vi "StandAloneApp_old.vi"() -> ()   [LabVIEW 2016]
panel:
  in  "Code 3":string
  in  "Code 2":string="# write code here\n"
  in  "Code 1":string="'''\nThis example will make SPIKE smile.\n\nIt is a good getting started example\n'''\n\nimport hub   # allows you to use all the SPIKE specific comands\n\nhub.display.show(hub.Image.SMILE)   # display a smile\n\n# for more examples on using the display, select the help button and look at the SPIKE examples\n"
  in  "Tab Control":enum32{"IntroPage", "Choose", "Examples"}(tab)
  in  "MoveOn":bool
  in  "Examples":bool
  in  "Blank":bool
  in  "W1.1 2":cluster{"Window Name":string, "Window1":bool}={"Window Name"="Select", "Window1"=FALSE}
  in  "W1.1 3":cluster{"Window Name":string, "Window1":bool}={"Window Name"="Select", "Window1"=FALSE}
  in  "W1.1":cluster{"Window Name":string, "Window1":bool}={"Window Name"="Select", "Window1"=FALSE}
  in  "Connections":enum32{"window 1", "window 2", "window 3"}(tab)
  in  "Device 3":bool
  in  "Device 2":bool
  in  "Device 1":bool
  in  "# Devices":enum32{"Page 1", "Page 2", "Page 3"}(tab)
  out "Description":string="This example will make SPIKE smile.\n\nIt is a good getting started example"
  out "Name":string="Smile"
  out "image":picture
  in  "Open Example":bool
  in  "Listbox":i32(listbox)
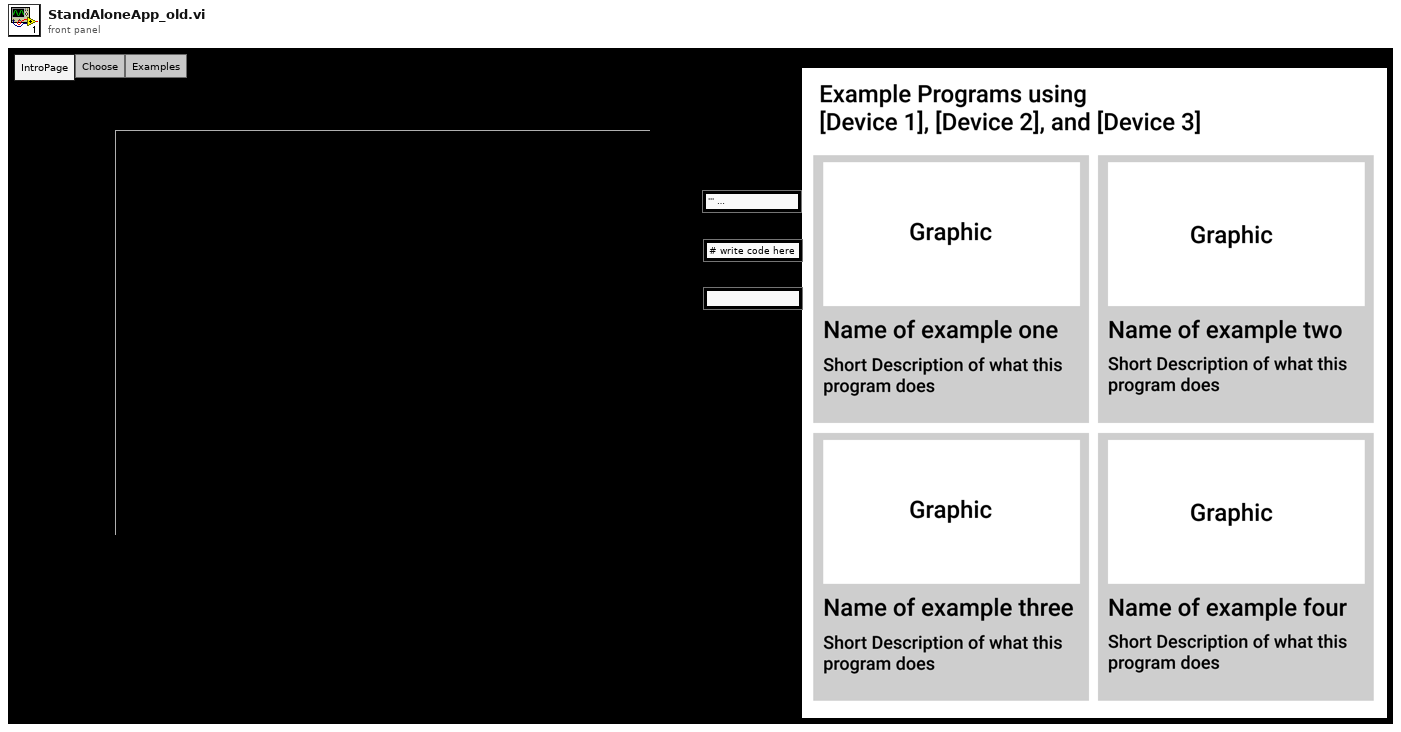
[diagram p1: front panel]
types:
  T1 = enum32{"Invalid", "Standard", "Closed", "Hidden", "Minimized", "Maximized"}
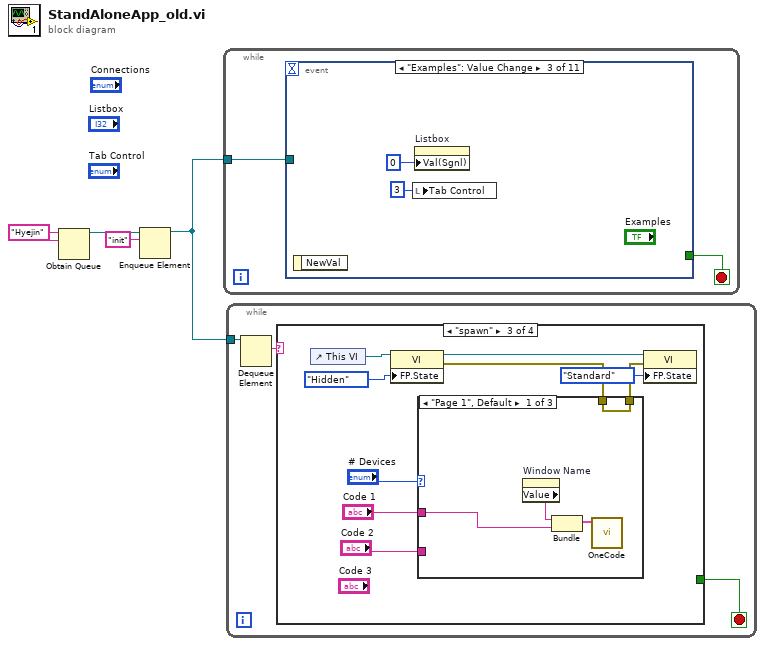
[diagram p0: block diagram]
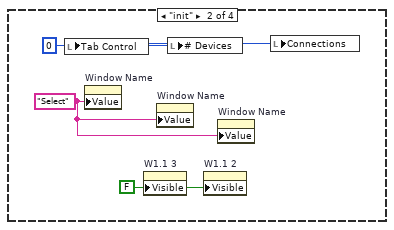
[diagram p3: hidden frame]
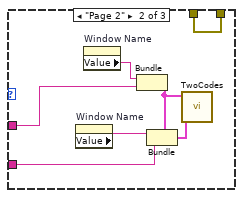
[diagram p4: hidden frame]
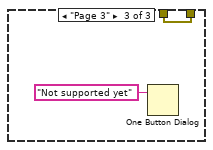
[diagram p5: hidden frame]
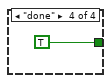
[diagram p6: hidden frame]
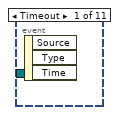
[diagram p7: hidden frame]
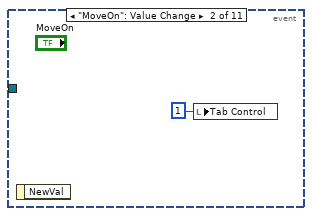
[diagram p8: hidden frame]
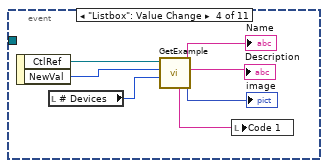
[diagram p9: hidden frame]
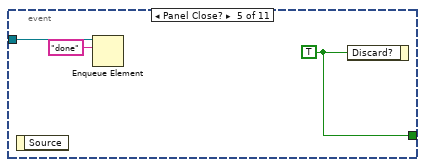
[diagram p10: hidden frame]
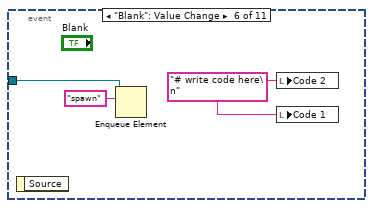
[diagram p11: hidden frame]
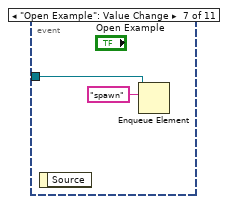
[diagram p12: hidden frame]
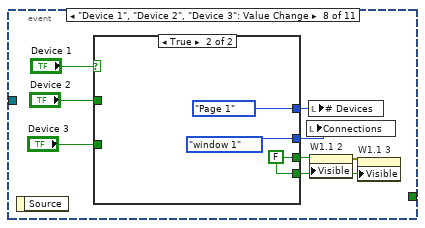
[diagram p13: hidden frame]
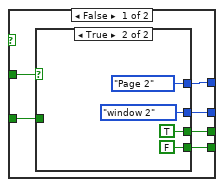
[diagram p14: hidden frame]
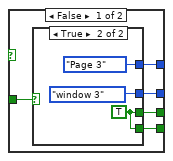
[diagram p15: hidden frame]
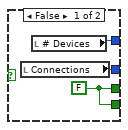
[diagram p16: hidden frame]
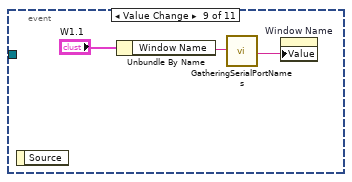
[diagram p17: hidden frame]
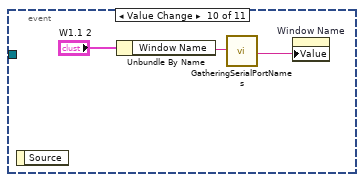
[diagram p18: hidden frame]
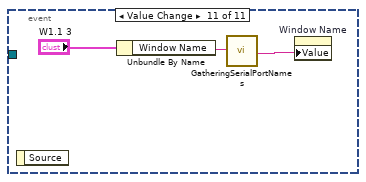
[diagram p19: hidden frame]
diagram:
  w1 = "Hyejin" ("name (unnamed)")
  n1 = Obtain Queue(name (unnamed)=w1, element data type=w1) -> (queue out=w4:refnum<queue>)  [unwired: 3 in, 2 out]
  n2 = Enqueue Element(queue=w4, element="init") -> (queue out=w2:refnum<queue>)  [unwired: 2 in, 2 out]
  n3 = while {
    tunnel: w2 -> [w5]
    stop <- w6 stop-if-true
    n4 = event shown="[2] \"Examples\": Value Change" {
      selector: _ -> [_ _ _ _ _ _ _ _ _ _ _]
      dyn-events: _ -> [_ _ _ _ _ _ _ _ _ _ _]
      timeout: _ -> [_ _ _ _ _ _ _ _ _ _ _]
      tunnel: [_ _ _ _ w19 _ _ _ _ _ _] -> w6
      tunnel: w5 -> [_ _ _ _ w17 w21 w23 _ _ _ _]
      event Timeout {
        n5 = event-data() -> ()  [unwired: 1 in, 3 out]
      }
      event "MoveOn": Value Change {
        n6 = event-data() -> ()  [unwired: 1 in, 1 out]
        n7 = local write "Tab Control"(1) -> ()
      }
      event "Examples": Value Change {
        n8 = event-data() -> ()  [unwired: 1 in, 1 out]
        n9 = local write "Tab Control"(3) -> ()
        n10 = property on="Listbox" class="LstBox (strict)"("Val(Sgnl)"=0 ("Listbox")) -> ()  [unwired: 2 in, 2 out]
      }
      event "Listbox": Value Change {
        n11 = event-data() -> ("CtlRef"=w15:refnum<vi>, "NewVal"=w14:i32)  [unwired: 1 in]
        n12 = local read "# Devices"() -> (w16:enum32{"Page 1", "Page 2", "Page 3"})
        n13 = call "GetExample.vi"("# Devices"=w16, "Listbox"=w14, "ListBox in"=w15) -> ("image"=→"image":picture, "description"=→"Description":string, "name"=→"Name":string, "Python"=w10:string)  [unwired: 5 in]
        n14 = local write "Code 1"(w10) -> ()
      }
      event Panel Close? {
        w19 = TRUE ("Discard?")
        n15 = event-data() -> ()  [unwired: 1 in, 1 out]
        n16 = Enqueue Element(queue=w17, element="done") -> ()  [unwired: 2 in, 3 out]
        n17 = event-data("Discard?"=w19) -> ()  [unwired: 1 in, 1 out]
      }
      event "Blank": Value Change {
        w20 = "# write code here\n" ("Code 2")
        n18 = event-data() -> ()  [unwired: 1 in, 1 out]
        n19 = Enqueue Element(queue=w21, element="spawn") -> ()  [unwired: 2 in, 3 out]
        n20 = local write "Code 2"(w20) -> ()
        n21 = local write "Code 1"(w20) -> ()
      }
      event "Open Example": Value Change {
        n22 = event-data() -> ()  [unwired: 1 in, 1 out]
        n23 = Enqueue Element(queue=w23, element="spawn") -> ()  [unwired: 2 in, 3 out]
      }
      event "Device 1", "Device 2", "Device 3": Value Change {
        n24 = event-data() -> ()  [unwired: 1 in, 1 out]
        n25 = case shown="True" "Device 1" {
          tunnel: [w38 enum32{"Page 1", "Page 2", "Page 3"}."Page 1" ("# Devices")] -> w32
          tunnel: "Device 2" -> [w37 _]
          tunnel: "Device 3" -> [w36 _]
          tunnel: [w35 enum32{"window 1", "window 2", "window 3"}."window 1" ("Connections 2")] -> w28
          tunnel: [w34 w54] -> w26
          tunnel: [w33 w54] -> w25
          frame False {
            n26 = case shown="True" w37 {
              tunnel: [w43 enum32{"Page 1", "Page 2", "Page 3"}."Page 2" ("# Devices")] -> w38
              tunnel: w36 -> [w42 _]
              tunnel: [w41 enum32{"window 1", "window 2", "window 3"}."window 2" ("Connections 2")] -> w35
              tunnel: [w40 TRUE ("Visible")] -> w34
              tunnel: [w39 FALSE ("Visible")] -> w33
              frame False {
                n27 = case shown="True" w42 {
                  tunnel: [w46 enum32{"Page 1", "Page 2", "Page 3"}."Page 3" ("# Devices")] -> w43
                  tunnel: [w45 enum32{"window 1", "window 2", "window 3"}."window 3" ("Connections 2")] -> w41
                  tunnel: [w44 w47] -> w40
                  tunnel: [w44 w47] -> w39
                  frame False {
                    w44 = FALSE ("Visible")
                    n28 = local read "Connections"() -> (w45:enum32{"window 1", "window 2", "window 3"})
                    n29 = local read "# Devices"() -> (w46:enum32{"Page 1", "Page 2", "Page 3"})
                  }
                  frame True {
                    w47 = TRUE ("Visible")
                  }
                }
              }
              frame True {
              }
            }
          }
          frame True {
            w54 = FALSE ("Visible")
          }
        }
        n30 = local write "Connections"(w28) -> ()
        n31 = local write "# Devices"(w32) -> ()
        n32 = property on="W1.1 2" class="Clust"("Visible"=w26) -> (error out=w27:errorcluster)  [unwired: 2 in, 1 out]
        n33 = property on="W1.1 3" class="Clust"(error in=w27, "Visible"=w25) -> ()  [unwired: 1 in, 2 out]
      }
      event "W1.1.Window1": Value Change {
        n34 = event-data() -> ()  [unwired: 1 in, 1 out]
        n35 = Unbundle By Name("W1.1") -> ("Window Name"=w58:string)
        n36 = call "GatheringSerialPortNames.vi"("old Name"=w58) -> ("name"=w57:string)  [unwired: 10 in]
        n37 = property on="Window Name" class="Str"("Value"=w57) -> ()  [unwired: 2 in, 2 out]
      }
      event "W1.1 2.Window1": Value Change {
        n38 = event-data() -> ()  [unwired: 1 in, 1 out]
        n39 = Unbundle By Name("W1.1 2") -> ("Window Name"=w62:string)
        n40 = call "GatheringSerialPortNames.vi"("old Name"=w62) -> ("name"=w60:string)  [unwired: 10 in]
        n41 = property on="Window Name" class="Str"("Value"=w60) -> ()  [unwired: 2 in, 2 out]
      }
      event "W1.1 3.Window1": Value Change {
        n42 = event-data() -> ()  [unwired: 1 in, 1 out]
        n43 = Unbundle By Name("W1.1 3") -> ("Window Name"=w65:string)
        n44 = call "GatheringSerialPortNames.vi"("old Name"=w65) -> ("name"=w63:string)  [unwired: 10 in]
        n45 = property on="Window Name" class="Str"("Value"=w63) -> ()  [unwired: 2 in, 2 out]
      }
    }
  }
  n46 = while {
    tunnel: w2 -> [w67]
    stop <- w66 stop-if-true
    n47 = Dequeue Element(queue=w67) -> (element=w68:string)  [unwired: 2 in, 3 out]
    n48 = case shown="\"spawn\"" w68 {
      tunnel: [_ _ _ TRUE ("Discard?")] -> w66
      frame Default {
      }
      frame "init" {
        w69 = FALSE ("Visible")
        w70 = "Select" ("Value")
        w71 = 0
        n49 = local write "Tab Control"(w71) -> ()
        n50 = property on="Window Name" class="Str"("Value"=w70) -> ()  [unwired: 2 in, 2 out]
        n51 = property on="W1.1 3" class="Clust"("Visible"=w69) -> ()  [unwired: 2 in, 2 out]
        n52 = property on="Window Name" class="Str"("Value"=w70) -> ()  [unwired: 2 in, 2 out]
        n53 = local write "# Devices"(w71) -> ()
        n54 = property on="W1.1 2" class="Clust"("Visible"=w69) -> ()  [unwired: 2 in, 2 out]
        n55 = property on="Window Name" class="Str"("Value"=w70) -> ()  [unwired: 2 in, 2 out]
        n56 = local write "Connections"(w71) -> ()
      }
      frame "spawn" {
        n57 = control-ref of="This VI"() -> (w77:refnum<vi>)
        n58 = property class="VI"(reference=w77, "FP.State"=T1."Hidden" ("Front Panel Window:State")) -> (reference out=w73:refnum<vi>, error out=w75:errorcluster)  [unwired: 1 in]
        n59 = case shown="\"Page 1\", Default" "# Devices" {
          tunnel: "Code 1" -> [w82 w87 _]
          tunnel: "Code 2" -> [_ w86 _]
          tunnel: [w81 w85 w92] -> w74
          tunnel: w75 -> [w81 w85 w92]
          frame "Page 1", Default {
            n60 = property on="Window Name" class="Str"() -> ("Value"=w83:string)  [unwired: 2 in, 2 out]
            n61 = Bundle("Value"=w83, "Code 1"=w82) -> (w84:cluster{"Value":string, "Code 1":string})  [unwired: 1 in]
            n62 = call "OneCode.vi"("Default"=w84) -> ()  [unwired: 11 in]
          }
          frame "Page 2" {
            n63 = property on="Window Name" class="Str"() -> ("Value"=w90:string)  [unwired: 2 in, 2 out]
            n64 = property on="Window Name" class="Str"() -> ("Value"=w91:string)  [unwired: 2 in, 2 out]
            n65 = Bundle("Value"=w91, "Code 1"=w87) -> (w89:cluster{"Value":string, "Code 1":string})  [unwired: 1 in]
            n66 = Bundle(cluster=w89, "Value"=w90, "Code 1"=w86) -> (w88:cluster{"Value":string, "Code 1":string})
            n67 = call "TwoCodes.vi"("Backpack"=w88, "Spike"=w89) -> ()  [unwired: 10 in]
          }
          frame "Page 3" {
            n68 = One Button Dialog(message="Not supported yet") -> ()  [unwired: 1 in, 1 out]
          }
        }
        n69 = property class="VI"(reference=w73, error in=w74, "FP.State"=T1."Standard" ("Front Panel Window:State")) -> ()  [unwired: 2 out]
      }
      frame "done" {
      }
    }
  }
